vi "load_class-class.vi"(8 "error in (no error)":errorcluster, 11 "class":refnum<class "v1.lvclass">) -> (0 "error out":errorcluster)   [LabVIEW 2015, in "lv-dialog.lvlib" / "v1.lvlib"]
uses:
  v1.lvlib
  class/v1.lvclass
  private/_controls/fg_command.ctl
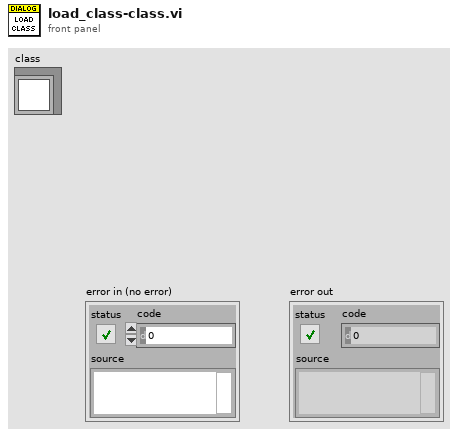
[diagram p1: front panel]
types:
  T1 = typedef "lv-dialog.lvlib/v1.lvlib/fg_command.ctl" = enum16{"null", "initialize", "read", "write", "shutdown"}
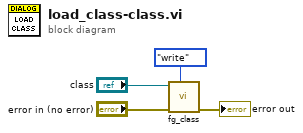
[diagram p0: block diagram]
diagram:
  n1 = call "fg_class.vi"("fg_command"=fg_command."write", "error in (no error)"="error in (no error)", "class in"="class") -> ("error out"=→"error out":errorcluster)  [unwired: 7 in, 1 out]
